vi "niScope Initialize With Options.vi"(0 "resource name":refnum<k15>="DAQ::1", 5 "id query":bool, 7 "option string":string="Simulate=0,RangeCheck=1,Cache=1", 9 "reset device":bool=TRUE, 11 "error in":errorcluster) -> (4 "instrument handle":refnum<k15>, 15 "error out":errorcluster)   [LabVIEW 2011]
doc: "Performs the following initialization actions:\n\n-Creates a new IVI instrument driver and optionally sets the initial state of the following session properties: Range Check, Cache, Simulate, Record Value Coercions.\n\n-Opens a session to the device that you specify in the resource name parameter.\n\n-Resets the instrument to a known state if the reset device parameter is set to TRUE; refer to niScope Reset for the default state of each digitizer.\n\n-Queries the instrument ID and verifies that it is valid for this instrument driver if the id query parameter is set to TRUE.\n\n-Returns an instrument handle that you use to identify the instrument in all subsequent instrument driver VI calls."
uses:
  niScope_32.dll
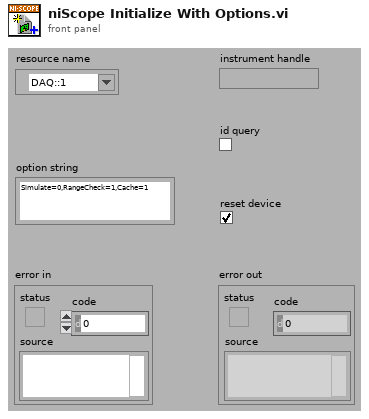
[diagram p1: front panel]
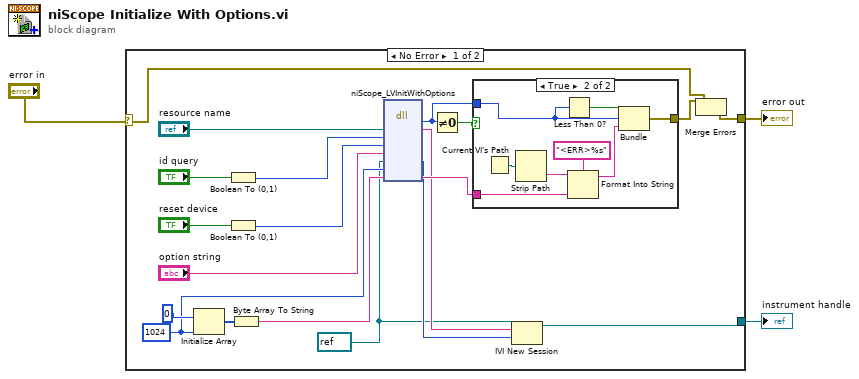
[diagram p0: block diagram]
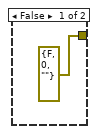
[diagram p2: hidden frame]
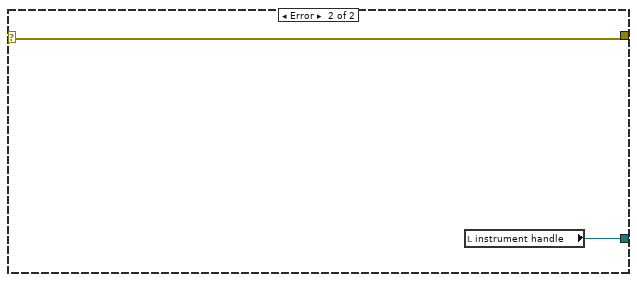
[diagram p3: hidden frame]
diagram:
  n1 = case shown="No Error" "error in" {
    selector: "error in" -> [w5 w33]
    tunnel: [w6 w33] -> w3
    tunnel: [w14 w34] -> w2
    frame No Error {
      w4 = refnum<k15> refnum
      w9 = 1024
      n2 = Initialize Array(0, w9) -> (w10:i32[])
      n3 = Boolean To (0,1)(Boolean="id query") -> (0, 1=w16:i16)
      n4 = Boolean To (0,1)(Boolean="reset device") -> (0, 1=w15:i16)
      n5 = Byte Array To String(unsigned byte array=w10) -> (string=w8:string)
      n6 = dll-call lib="niScope_*.*" fn="niScope_LVInitWithOptions"("resourceName"="resource name", "IDQuery"=w16, "resetDevice"=w15, "optionString"="option string", "instrument handle"=w4, "error buffer size"=w9, "error buffer"=w8) -> ("status"=w18:i32, "resourceName"=w13:string, "instrument handle"=w12:u32, "error buffer"=w17:string)  [unwired: 7 in, 2 out]
      n7 = Not Equal To 0?(x=w18) -> (x != 0?=w19:bool)
      n8 = case shown="True" w19 {
        tunnel: w17 -> [_ w32]
        tunnel: w18 -> [_ w27]
        tunnel: [cluster{bool, "status":i32, string} {FALSE, "status"=0, ""} w25] -> w7
        frame False {
        }
        frame True {
          n9 = Current VI's Path() -> (path=w30:path)
          n10 = Strip Path(path=w30) -> (name=w29:string)  [unwired: 1 out]
          n11 = Less Than 0?(x=w27) -> (x < 0?=w26:bool)
          n12 = Format Into String(format string="<ERR>%s", initial string=w29, w32) -> (resulting string=w28:string)  [unwired: 1 in, 1 out]
          n13 = Bundle(w26, "status"=w27, w28) -> (w25:cluster{bool, "status":i32, string})  [unwired: 1 in]
        }
      }
      n14 = IVI New Session(9:w12, 10:w13, 11:w4) -> (3:w14:refnum<k15>)
      n15 = Merge Errors(w5, w7) -> (w6:errorcluster)
    }
    frame Error {
      n16 = local read "instrument handle"() -> (w34:refnum<k15>)
    }
  }
  "error out" <- w3
  "instrument handle" <- w2
